vi "TR_ManageMenu.vi"(8 "error in (no error)":errorcluster, 11 "Menu in":refnum<class "Menu.lvclass">) -> (0 "error out":errorcluster)   [LabVIEW 2021, in "Menu.lvlib" / "Menu.lvclass"]
uses:
  Menu.lvclass
  Menu.lvclass/Menu.ctl
  687d16a6-6148-407a-a2d8-39ae7b2e2ec5.vi
  InputDevice/src/Mouse/Mouse.lvclass
  InputDevice/src/Keyboard/Keyboard.lvclass
  <vilib>/Utility/miscctls.llb/LVPoint32TypeDef.ctl
  <vilib>/event_ctls.llb/usereventprio.ctl
  90e311d3-1a3a-4c58-ba76-d298bb06b0d5.vi
  VIActivation/VIActivation.lvclass
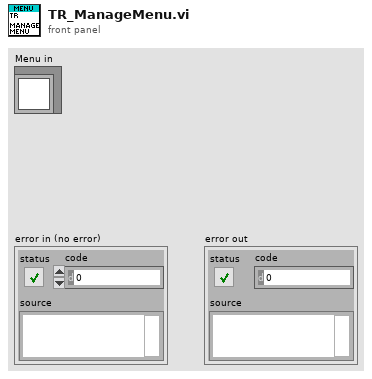
[diagram p1: front panel]
types:
  T1 = typedef "LVPoint32TypeDef.ctl" = cluster{"Horizontal":i32, "Vertical":i32}
  T2 = typedef "usereventprio.ctl" = enum32{"high priority", "normal priority"}
  T3 = cluster{"Mouse":refnum<event-registration>, "Keyboard":refnum<event-registration>, "Event Registration Refnum":refnum<event-registration>, "VIActivation":refnum<event-registration>}
  T4 = cluster{"left":i16, "top":i16, "right":i16, "bottom":i16}
  T5 = enum16{"0", "1", "2", "3", "4", "5", "6", "7", "8", "9", "A", "B", "C", "D", "E", "F", "G", "H", "I", "J", "K", "L", "M", "N", "O", "P", "Q", "R", "S", "T", "U", "V", "W", "X", "Y", "Z", "F1", "F2", "F3", "F4", "F5", "F6", "F7", "F8", "F9", "F10", "F11", "F12", "F13", "F14", "F15", "ADD", "BACK", "BACKSLASH", "CAPITAL", "COMMA", "DECIMAL", "DELETE", "DIVIDE", "DOWN", "END", "EQUALS", "ESCAPE", "GRAVE (`)", "HOME", "INSERT", "LBRACKET", "LCONTROL", "LEFT", "L ALT", "LSHIFT", "LWIN", "MINUS", "MULTIPLY", "NEXT", "NUMLOCK", "NUMPAD_0", "NUMPAD_1", "NUMPAD_2", "NUMPAD_3", "NUMPAD_4", "NUMPAD_5", "NUMPAD_6", "NUMPAD_7", "NUMPAD_8", "NUMPAD_9", "PAUSE", "PERIOD", "PRIOR (PG UP)", "RBRACKET", "RCONTROL", "RETURN", "RIGHT", "R ALT", "RSHIFT", "RWIN", "SCROLL", "SEMICOLON", "SLASH", "SPACE", "SUBTRACT", "TAB", "UP", "ENTER (num pad)", "' (quote)"}[]
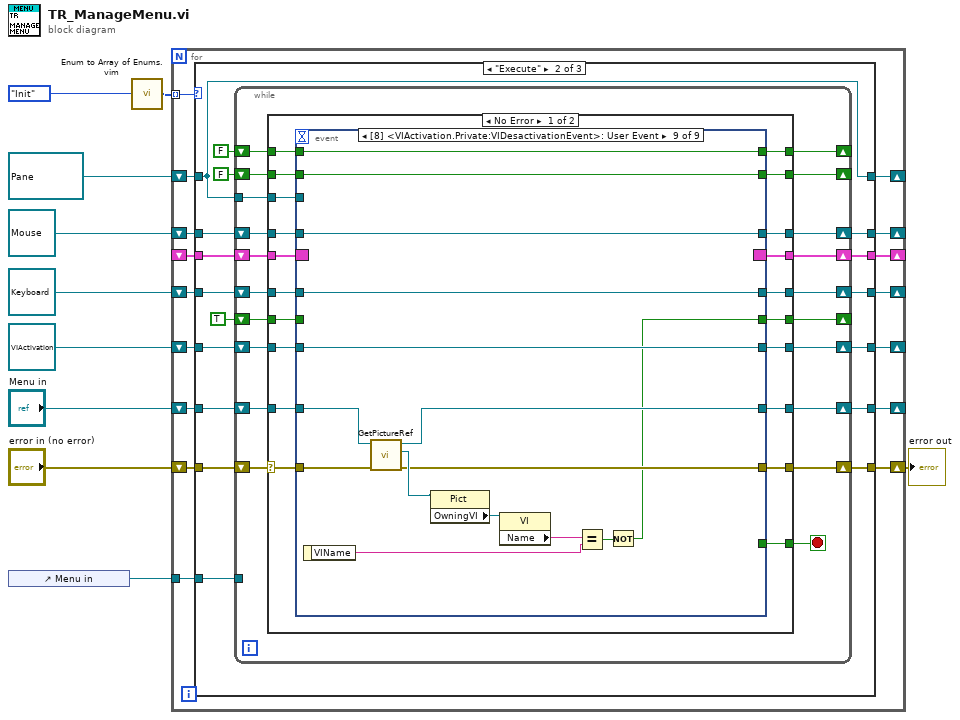
[diagram p0: block diagram]
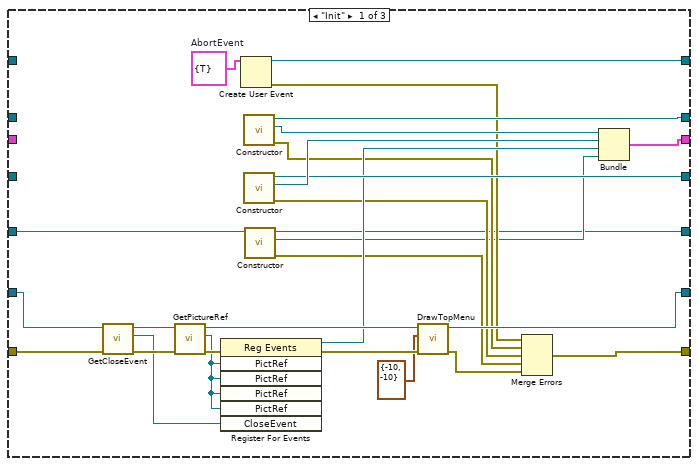
[diagram p2: hidden frame]
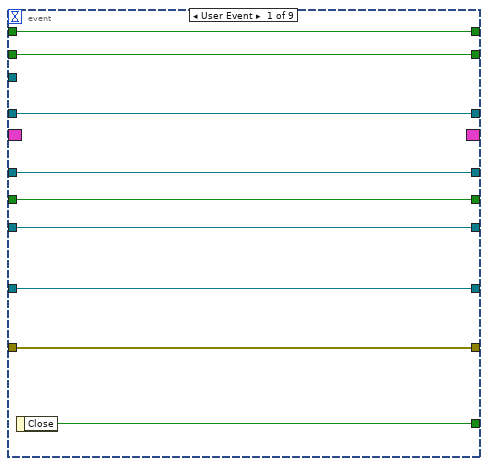
[diagram p3: hidden frame]
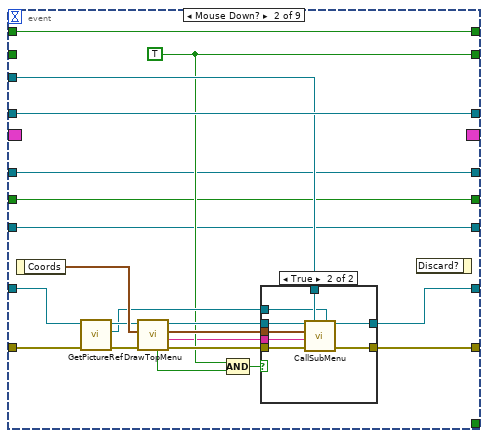
[diagram p4: hidden frame]
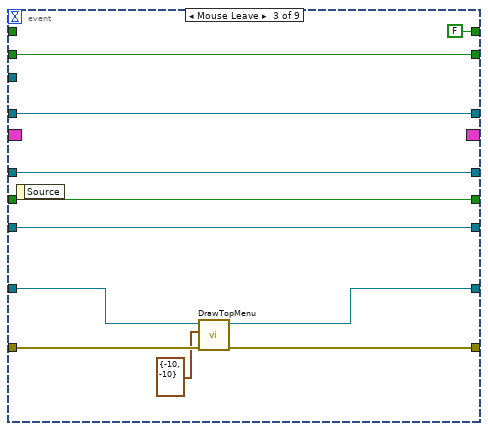
[diagram p6: hidden frame]
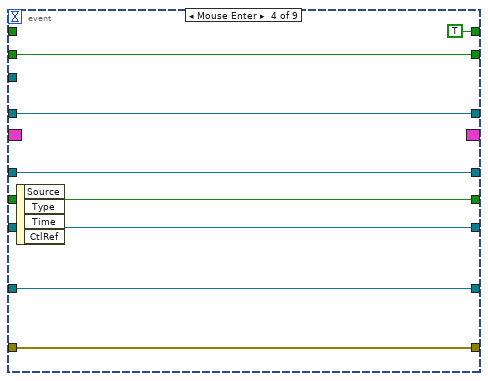
[diagram p7: hidden frame]
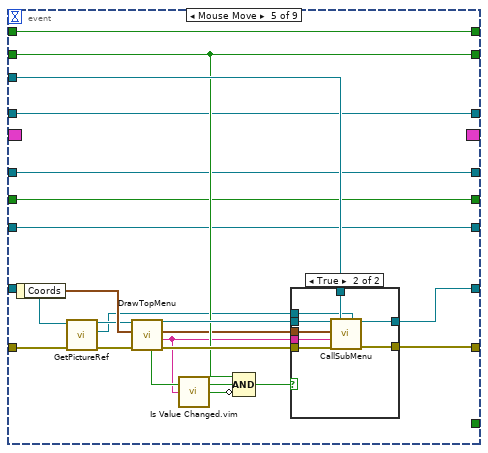
[diagram p8: hidden frame]
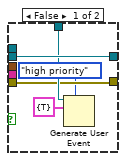
[diagram p9: hidden frame]
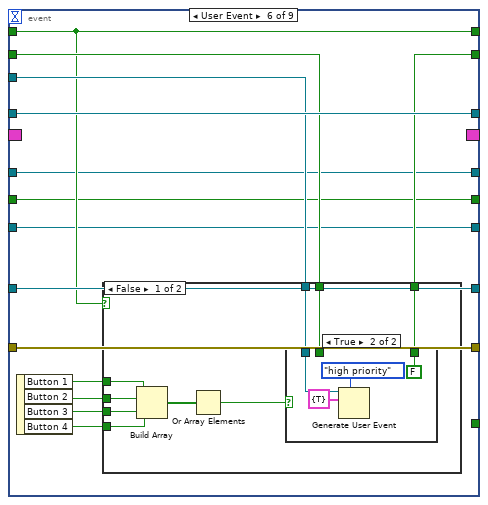
[diagram p10: hidden frame]
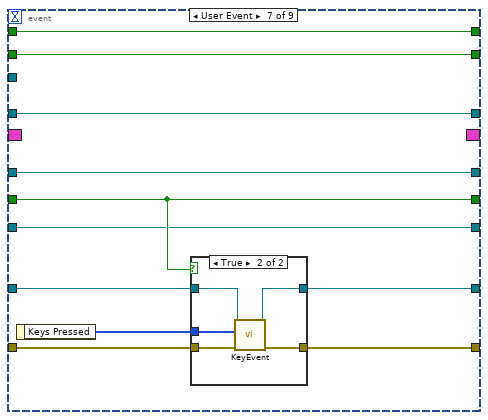
[diagram p13: hidden frame]
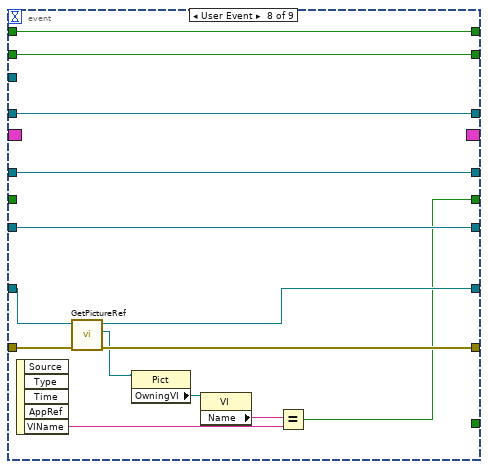
[diagram p15: hidden frame]
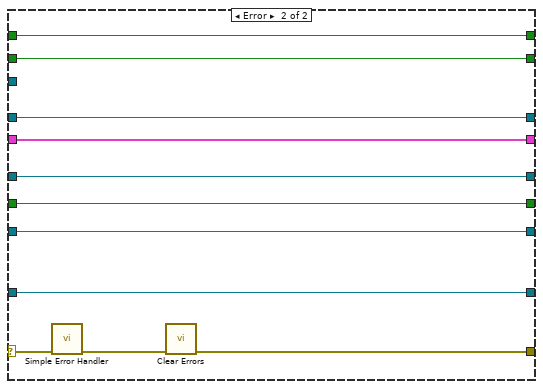
[diagram p16: hidden frame]
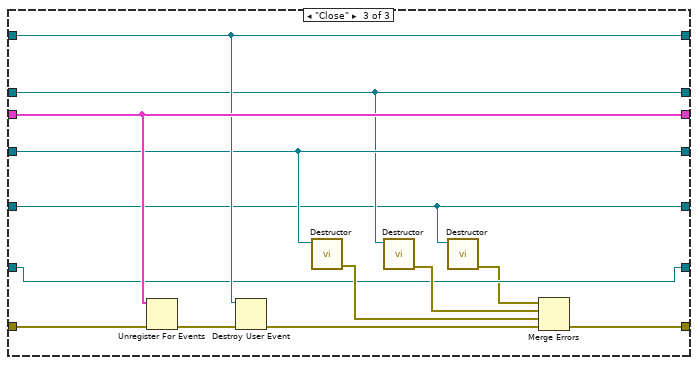
[diagram p17: hidden frame]
diagram:
  n1 = control-ref of="Menu in"() -> (w10:refnum<vi>)
  n2 = call "Enum to Array of Enums.vim"("enum"=enum16{"Init", "Execute", "Close"}."Init") -> ("array of enums"=w8:enum16{"Init", "Execute", "Close"}[])
  n3 = for {
    tunnel: w10 -> [w24]
    shift-right: [w16] -> _
    shift-left: refnum<class "Mouse.lvclass"> refnum ("Mouse out") -> [w15]
    shift-right: [w20] -> _
    shift-left: _ -> [w26]
    shift-right: [w18] -> w7
    shift-left: "error in (no error)" -> [w25]
    shift-right: [w17] -> _
    shift-left: refnum<class "Keyboard.lvclass"> refnum ("Keyboard out") -> [w22]
    tunnel: w8 -> [w21] mode=indexing
    shift-right: [w19] -> _
    shift-left: refnum<user-event> refnum ("AbortEvent") -> [w23]
    shift-right: [w13] -> _
    shift-left: "Menu in" -> [w14]
    shift-right: [w12] -> _
    shift-left: refnum<class "VIActivation.lvclass"> refnum ("VIActivation in") -> [w11]
    n4 = case shown="\"Execute\"" w21 {
      tunnel: [w51 w60 w296] -> w16
      tunnel: w26 -> [_ w71 w305]
      tunnel: [w52 w69 w305] -> w20
      tunnel: w25 -> [w40 w68 w304]
      tunnel: [w36 w67 w299] -> w18
      tunnel: w24 -> [_ w66 _]
      tunnel: w23 -> [_ w62 w302]
      tunnel: w22 -> [_ w64 w300]
      tunnel: [w48 w63 w300] -> w17
      tunnel: [w53 w62 w302] -> w19
      tunnel: w15 -> [_ w61 w296]
      tunnel: w14 -> [w42 w58 w295]
      tunnel: [w39 w59 w295] -> w13
      tunnel: [w30 w55 w294] -> w12
      tunnel: w11 -> [w27 w56 w294]
      frame "Init" {
        w54 = cluster{"Abort":bool} {"Abort"=TRUE}  # AbortEvent
        n5 = call "GetCloseEvent.vi"("error in (no error)"=w40, "Menu in"=w42) -> ("error out"=w45:errorcluster, "CloseEvent"=w37:refnum<user-event>, "Menu out"=w44:refnum<class "Menu.lvclass">)  [unwired: 7 in]
        n6 = call "GetPictureRef.vi"("error in (no error)"=w45, "Menu in"=w44) -> ("error out"=w46:errorcluster, "PictRef"=w32:refnum<vi>, "Menu out"=w47:refnum<class "Menu.lvclass">)  [unwired: 7 in]
        n7 = register-events ("RegEvents")(error in=w46, w32, w32, w32, w32, w37) -> (reference out=w38:refnum<event-registration>, error out=w43:errorcluster)  [unwired: 1 in]
        n8 = Create User Event(user event datatype=w54) -> (user event=w53:refnum<user-event>, error out=w33:errorcluster)  [unwired: 1 in]
        n9 = call "Constructor.vi"() -> ("error out"=w34:errorcluster, "Mouse"=w50:refnum<event-registration>, "Mouse out"=w51:refnum<class "Mouse.lvclass">)  [unwired: 9 in]
        n10 = call "Constructor.vi"() -> ("error out"=w35:errorcluster, "Keyboard"=w49:refnum<event-registration>, "Keyboard out"=w48:refnum<class "Keyboard.lvclass">)  [unwired: 9 in]
        n11 = call "Constructor.vi"("VIActivation in"=w27) -> ("error out"=w28:errorcluster, "VIActivation"=w31:refnum<event-registration>, "VIActivation out"=w30:refnum<class "VIActivation.lvclass">)  [unwired: 8 in]
        n12 = call "DrawTopMenu.vi"("error in (no error)"=w43, "Coords"=T1 {"Horizontal"=-10, "Vertical"=-10}, "Menu in"=w47) -> ("error out"=w29:errorcluster, "Menu out"=w39:refnum<class "Menu.lvclass">)  [unwired: 4 in, 3 out]
        n13 = Merge Errors(w33, w34, w35, w28, w29) -> (w36:errorcluster)
        n14 = Bundle("Mouse"=w50, "Keyboard"=w49, "Event Registration Refnum"=w38, "VIActivation"=w31) -> (w52:T3)  [unwired: 1 in]
      }
      frame "Execute" {
        n15 = while {
          shift-right: [w88] -> w59
          shift-left: w58 -> [w91]
          tunnel: w62 -> [w85]
          shift-right: [w83] -> _
          shift-left: FALSE -> [w84]
          shift-right: [w81] -> w60
          shift-left: w61 -> [w82]
          shift-right: [w86] -> w69
          shift-left: w71 -> [w87]
          shift-right: [w89] -> w67
          shift-left: w68 -> [w90]
          tunnel: w66 -> [_]
          shift-right: [w78] -> _
          shift-left: FALSE -> [w79]
          shift-right: [w76] -> w63
          shift-left: w64 -> [w77]
          shift-right: [w74] -> _
          shift-left: TRUE -> [w75]
          shift-right: [w72] -> w55
          shift-left: w56 -> [w73]
          stop <- w80 stop-if-true
          n16 = case shown="No Error" w90 {
            selector: w90 -> [w110 w292]
            tunnel: w91 -> [w111 w291]
            tunnel: [w109 w289] -> w89
            tunnel: [w108 w291] -> w88
            tunnel: w87 -> [w107 w288]
            tunnel: [w106 w288] -> w86
            tunnel: w85 -> [w105 _]
            tunnel: w84 -> [w104 w287]
            tunnel: [w103 w287] -> w83
            tunnel: w82 -> [w102 w286]
            tunnel: [w101 w286] -> w81
            tunnel: [w100 _] -> w80
            tunnel: w79 -> [w99 w285]
            tunnel: [w98 w285] -> w78
            tunnel: w77 -> [w97 w284]
            tunnel: [w96 w284] -> w76
            tunnel: w75 -> [w95 w283]
            tunnel: [w94 w283] -> w74
            tunnel: w73 -> [w93 w282]
            tunnel: [w92 w282] -> w72
            frame No Error {
              n17 = event shown="[8] <VIActivation.Private:VIDesactivationEvent>: User Event" {
                selector: w107 -> [_ _ _ _ _ _ _ _ _]
                dyn-events: [_ _ _ _ _ _ _ _ _] -> w106
                timeout: _ -> [_ _ _ _ _ _ _ _ _]
                tunnel: w111 -> [w120 w132 w162 w169 w178 w219 w241 w259 w270]
                tunnel: w110 -> [w117 w129 w160 w170 w175 w212 w239 w261 w273]
                tunnel: [w117 w140 w159 w170 w189 w212 w238 w260 w272] -> w109
                tunnel: [w120 w138 w161 w169 w191 w219 w240 w258 w271] -> w108
                tunnel: w105 -> [_ w134 _ _ w188 w213 _ _ _]
                tunnel: w104 -> [w119 _ w156 w168 w186 w210 w245 w266 w281]
                tunnel: [w119 w127 w156 w168 w186 w211 w245 w266 w281] -> w103
                tunnel: w102 -> [w118 w137 w158 w167 w185 w218 w244 w265 w280]
                tunnel: [w118 w137 w158 w167 w185 w218 w244 w265 w280] -> w101
                tunnel: [w116 _ _ _ _ _ _ _ _] -> w100
                tunnel: w99 -> [w115 w124 _ _ w174 w209 w243 w264 w279]
                tunnel: [w115 w124 FALSE TRUE w174 w209 w243 w264 w279] -> w98
                tunnel: w97 -> [w114 w123 w154 w165 w173 w208 w242 w263 w278]
                tunnel: [w114 w123 w154 w165 w173 w208 w242 w263 w278] -> w96
                tunnel: w95 -> [w113 w122 w153 w164 w172 w207 w236 _ _]
                tunnel: [w113 w122 w153 w164 w172 w207 w236 w253 w267] -> w94
                tunnel: [w112 w121 w152 w163 w171 w206 w235 w262 w277] -> w92
                tunnel: w93 -> [w112 w121 w152 w163 w171 w206 w235 w262 w277]
                event User Event {
                  n18 = event-data() -> ("Close"=w116:bool)  [unwired: 1 in]
                }
                event Mouse Down? {
                  w127 = TRUE
                  n19 = event-data() -> ("Coords"=w136:T1)  [unwired: 1 in]
                  n20 = call "GetPictureRef.vi"("error in (no error)"=w129, "Menu in"=w132) -> ("error out"=w130:errorcluster, "PictRef"=w131:refnum<vi>, "Menu out"=w133:refnum<class "Menu.lvclass">)  [unwired: 7 in]
                  n21 = call "DrawTopMenu.vi"("error in (no error)"=w130, "Coords"=w136, "Menu in"=w133) -> ("error out"=w141:errorcluster, "Selected Tag"=w125:string, "Selected Area"=w135:T4, "Menu out"=w139:refnum<class "Menu.lvclass">, "SubMenu"=w126:bool)  [unwired: 4 in]
                  n22 = Compound Arithmetic op=AND(w127, w126) -> (w128:bool)
                  n23 = case shown="True" w128 {
                    tunnel: w125 -> [_ w151]
                    tunnel: w135 -> [_ w150]
                    tunnel: w141 -> [w142 w149]
                    tunnel: [w142 w148] -> w140
                    tunnel: w139 -> [w143 w147]
                    tunnel: [w143 w146] -> w138
                    tunnel: w134 -> [_ w145]
                    tunnel: w131 -> [_ w144]
                    frame False {
                    }
                    frame True {
                      n24 = call "CallSubMenu.vi"("Menu in"=w147, "User Event"=w145, "CtrlRef"=w144, "Selected Area"=w150, "Selected Tag"=w151, "error in (no error)"=w149) -> ("Menu out"=w146:refnum<class "Menu.lvclass">, "error out"=w148:errorcluster)  [unwired: 8 in]
                    }
                  }
                  n25 = event-data() -> ()  [unwired: 2 in, 1 out]
                }
                event Mouse Leave {
                  n26 = event-data() -> ()  [unwired: 1 in, 1 out]
                  n27 = call "DrawTopMenu.vi"("error in (no error)"=w160, "Coords"=T1 {"Horizontal"=-10, "Vertical"=-10}, "Menu in"=w162) -> ("error out"=w159:errorcluster, "Menu out"=w161:refnum<class "Menu.lvclass">)  [unwired: 4 in, 3 out]
                }
                event Mouse Enter {
                  n28 = event-data() -> ()  [unwired: 1 in, 4 out]
                }
                event Mouse Move {
                  n29 = event-data() -> ("Coords"=w183:T1)  [unwired: 1 in]
                  n30 = call "GetPictureRef.vi"("error in (no error)"=w175, "Menu in"=w178) -> ("error out"=w176:errorcluster, "PictRef"=w177:refnum<vi>, "Menu out"=w179:refnum<class "Menu.lvclass">)  [unwired: 7 in]
                  n31 = call "DrawTopMenu.vi"("error in (no error)"=w176, "Coords"=w183, "Menu in"=w179) -> ("error out"=w190:errorcluster, "Selected Tag"=w184:string, "Selected Area"=w182:T4, "Menu out"=w192:refnum<class "Menu.lvclass">, "SubMenu"=w187:bool)  [unwired: 4 in]
                  n32 = call "Is Value Changed.vim"("value"=w184) -> ("changed or first call?"=w181:bool)
                  n33 = Compound Arithmetic op=AND(w186, w187, invert w181) -> (w180:bool)
                  n34 = case shown="True" w180 {
                    tunnel: w192 -> [w197 w205]
                    tunnel: [w197 w204] -> w191
                    tunnel: w190 -> [w194 w203]
                    tunnel: [w194 w202] -> w189
                    tunnel: w182 -> [_ w201]
                    tunnel: w184 -> [_ w200]
                    tunnel: w188 -> [w196 w199]
                    tunnel: w177 -> [_ w198]
                    frame False {
                      n35 = Generate User Event(priority (normal)=usereventprio."high priority", user event=w196, event data cluster=cluster{"Abort":bool} {"Abort"=TRUE} ("event data")) -> ()  [unwired: 1 in, 2 out]
                    }
                    frame True {
                      n36 = call "CallSubMenu.vi"("Menu in"=w205, "User Event"=w199, "CtrlRef"=w198, "Selected Area"=w201, "Selected Tag"=w200, "error in (no error)"=w203) -> ("Menu out"=w204:refnum<class "Menu.lvclass">, "error out"=w202:errorcluster)  [unwired: 8 in]
                    }
                  }
                }
                event User Event {
                  n37 = event-data() -> ("Button 1"=w217:bool, "Button 2"=w216:bool, "Button 3"=w215:bool, "Button 4"=w214:bool)  [unwired: 1 in]
                  n38 = case shown="False" w209 {
                    tunnel: w217 -> [w228 _]
                    tunnel: w216 -> [w227 _]
                    tunnel: w215 -> [w226 _]
                    tunnel: w214 -> [w225 _]
                    tunnel: w213 -> [w223 _]
                    tunnel: [w221 w234] -> w211
                    tunnel: w210 -> [w220 w234]
                    frame False {
                      n39 = Build Array(w228, w227, w226, w225) -> (w224:bool[])
                      n40 = Or Array Elements(Boolean array=w224) -> (logical OR=w222:bool)
                      n41 = case shown="True" w222 {
                        tunnel: w223 -> [_ w233]
                        tunnel: [w229 FALSE] -> w221
                        tunnel: w220 -> [w229 _]
                        frame False {
                        }
                        frame True {
                          n42 = Generate User Event(priority (normal)=usereventprio."high priority", user event=w233, event data cluster=cluster{"Abort":bool} {"Abort"=TRUE} ("event data")) -> ()  [unwired: 1 in, 2 out]
                        }
                      }
                    }
                    frame True {
                    }
                  }
                }
                event User Event {
                  n43 = event-data() -> ("Keys Pressed"=w237:T5)  [unwired: 1 in]
                  n44 = case shown="True" w236 {
                    tunnel: w241 -> [w247 w252]
                    tunnel: [w247 w251] -> w240
                    tunnel: w239 -> [w246 w250]
                    tunnel: [w246 w249] -> w238
                    tunnel: w237 -> [_ w248]
                    frame False {
                    }
                    frame True {
                      n45 = call "KeyEvent.vi"("error in (no error)"=w250, "Keys Pressed"=w248, "Menu in"=w252) -> ("error out"=w249:errorcluster, "Menu out"=w251:refnum<class "Menu.lvclass">)  [unwired: 7 in]
                    }
                  }
                }
                event User Event {
                  n46 = event-data() -> ("VIName"=w254:string)  [unwired: 1 in, 4 out]
                  n47 = call "GetPictureRef.vi"("error in (no error)"=w261, "Menu in"=w259) -> ("error out"=w260:errorcluster, "PictRef"=w257:refnum<vi>, "Menu out"=w258:refnum<class "Menu.lvclass">)  [unwired: 7 in]
                  n48 = property class="Pict"(reference=w257) -> ("OwningVI"=w256:refnum<vi>)  [unwired: 1 in, 2 out]
                  n49 = property class="VI"(reference=w256) -> ("Name"=w255:string)  [unwired: 1 in, 2 out]
                  n50 = Equal?(x=w255, y=w254) -> (x = y?=w253:bool)
                }
                event User Event {
                  n51 = event-data() -> ("VIName"=w269:string)  [unwired: 1 in]
                  n52 = call "GetPictureRef.vi"("error in (no error)"=w273, "Menu in"=w270) -> ("error out"=w272:errorcluster, "PictRef"=w276:refnum<vi>, "Menu out"=w271:refnum<class "Menu.lvclass">)  [unwired: 7 in]
                  n53 = property class="Pict"(reference=w276) -> ("OwningVI"=w275:refnum<vi>)  [unwired: 1 in, 2 out]
                  n54 = property class="VI"(reference=w275) -> ("Name"=w274:string)  [unwired: 1 in, 2 out]
                  n55 = Equal?(x=w274, y=w269) -> (x = y?=w268:bool)
                  n56 = Not(x=w268) -> (.not. x?=w267:bool)
                }
              }
            }
            frame Error {
              n57 = call <vilib>:"Simple Error Handler.vi"("error in (no error)"=w292) -> ("error out"=w290:errorcluster)  [unwired: 4 in, 4 out]
              n58 = call <vilib>:"Clear Errors.vi"("error in (no error)"=w290) -> ("error out"=w289:errorcluster)  [unwired: 5 in, 1 out]
            }
          }
        }
      }
      frame "Close" {
        n59 = Unregister For Events(event registration refnum=w305, error in=w304) -> (error out=w303:errorcluster)
        n60 = Destroy User Event(user event=w302, error in=w303) -> (error out=w301:errorcluster)
        n61 = call-dynamic "Destructor.vi"("Mouse in"=w300) -> ("error out"=w297:errorcluster)  [unwired: 10 in]
        n62 = call-dynamic "Destructor.vi"("Mouse in"=w296) -> ("error out"=w298:errorcluster)  [unwired: 10 in]
        n63 = call "Destructor.vi"("VIActivation in"=w294) -> ("error out"=w293:errorcluster)  [unwired: 10 in]
        n64 = Merge Errors(w293, w298, w297, w301) -> (w299:errorcluster)
      }
    }
  }
  "error out" <- w7
